vi "Load and Open All Items.vi"(8 "error in (no error)":errorcluster, 11 "Application Data in":T1) -> (0 "error out":errorcluster, 3 "Application Data out":T1)   [LabVIEW 2017, in "DSF Configuration Utility.lvlib"]
uses:
  DSF Configuration Utility.lvlib
  Application Data.ctl
  VeriStand/Data Sharing Custom Device/Source/Engine/DSF Core.lvlibp/Classes/Configuration/Configuration Session.lvclass
  View Mode.ctl
  Set UI Busy State.vi
  Item Tree/Load Subitems.vi
  VeriStand/Data Sharing Custom Device/Source/Engine/DSF Core.lvlibp/Classes/Configuration/Read All Item IDs.vi
  VeriStand/Data Sharing Custom Device/Source/Engine/DSF Core.lvlibp/Classes/Configuration/Read All Plugin IDs.vi
panel:
  # "App\nData"
  # "App\nData"
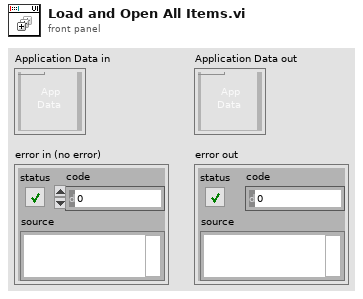
[diagram p1: front panel]
types:
  T1 = typedef "DSF Configuration Utility.lvlib/Application Data.ctl" = cluster{"Item Tree Control":refnum<vi>, "Value Tree Control":refnum<vi>, "DSF Refnum":refnum<class "Configuration Session.lvclass">, "Top-Level VI":refnum<vi>, "View State":T2, "menu reference":refnum<k9>}
  T2 = typedef "DSF Configuration Utility.lvlib/View Mode.ctl" = enum16{"Tree", "List"}
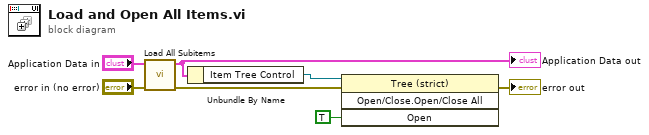
[diagram p0: block diagram]
diagram:
  n1 = call "Load All Subitems.vi"("error in (no error)"="error in (no error)", "Application Data in"="Application Data in") -> ("error out"=w1:errorcluster, "Application Data out"=w4:T1)  [unwired: 8 in]
  "Application Data out" <- w4
  n2 = Unbundle By Name(w4) -> ("Item Tree Control"=w6:refnum<vi>)
  n3 = invoke class="Tree (strict)" method="Open/Close.Open/Close All"(reference=w6, error in=w1, "Open"=TRUE ("Open?")) -> (error out=→"error out":errorcluster)  [unwired: 1 in, 3 out]
